vi "Read MC Analog In.vi"(8 "error in (no error)":errorcluster, 11 "channel":i32=2) -> (0 "error out":errorcluster, 3 "Voltage Input":dbl)   [LabVIEW 2016]
doc: "Reads a single point from the specified channel of the DAQ card.\nINPUTS:\n channel - channel number of the DAQ card, indexed from 0\nOUTPUT:\n datum - current value on the requested channel of the DAQ card\nPOTENTIAL ERRORS:\n Unspecified Labview Errors, 5009 (DAQ read error), 5010 (unknown DAQ type)"
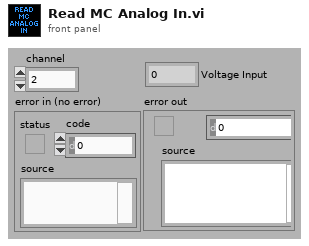
[diagram p1: front panel]
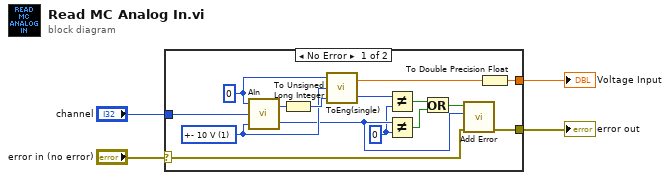
[diagram p0: block diagram]
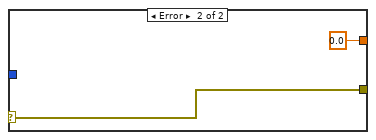
[diagram p2: hidden frame]
diagram:
  n1 = case shown="No Error" "error in (no error)" {
    selector: "error in (no error)" -> [w16 w21]
    tunnel: [w19 0.0] -> w4
    tunnel: "channel" -> [w18 _]
    tunnel: [w17 w21] -> w1
    frame No Error {
      w5 = 0 ("y")
      w7 = 1 items=["Not Programmable"=0, "+- 20 V"=27, "+- 10 V"=1, "+- 5 V"=2, "+- 4 V"=28, "+- 2.5 V"=3, "+- 2 V"=29, "+- 1.67 V"=4, "+- 1.25 V"=5, "+- 1 V"=6, "+- .625 V"=7, "+- .5 V"=8, "+- .25 V"=30, "+- .2 V"=31, "+- .1 V"=9, "+- .05 V"=10, "+- .01 V"=11, "+- .005 V"=12, "0 - 10 V"=13, "0 - 5 V"=14, "0 - 4 V"=36, "0 - 2.5 V"=15, "0 - 2 V"=16, "0 - 1.67 V"=17, "0 - 1.25 V"=18, "0 - 1 V"=19, "0 - .5 V"=32, "0 - .25 V"=33, "0 - .2 V"=34, "0 - .1 V"=20, "0 - .02 V"=35, "0 - .01 V"=21, "4 - 20 mA"=22, "2 - 10 mA"=23, "1 - 5 mA"=24, ".5 - 2.5 mA"=25, "0 - 20 mA"=26] ("Range")
      w15 = u32 0 ("BoardNum")
      n2 = call "AIn.VI"("Range"=w7, "Channel"=w18, "BoardNum"=w15) -> ("ErrCode"=w6:i32, "DataValue"=w14:u16)
      n3 = To Unsigned Long Integer(number=w14) -> (unsigned 32bit integer=w13:u32)
      n4 = call "ToEng(single).VI"("AD Data"=w13, "Range"=w7, "BoardNum (0)"=w15) -> ("ErrCode"=w11:i32, "Eng Units"=w12:sgl)
      n5 = Not Equal?(x=w11, y=w5) -> (x != y?=w10:bool)
      n6 = Not Equal?(x=w6, y=w5) -> (x != y?=w9:bool)
      n7 = Or(x=w10, y=w9) -> (x .or. y?=w8:bool)
      n8 = call "Add Error.vi"("error in (no error)"=w16, "error code (0)"=w6, "error?"=w8) -> ("error out"=w17:errorcluster)  [unwired: 8 in]
      n9 = To Double Precision Float(number=w12) -> (double precision float=w19:dbl)
    }
    frame Error {
    }
  }
  "Voltage Input" <- w4
  "error out" <- w1
